vi "stage.vi"(8 "error in (no error)":errorcluster, 9 "stage number":u64, 11 "simonMessages in":refnum<class "simonMessages.lvclass">) -> (0 "error out":errorcluster, 3 "simonMessages out":refnum<class "simonMessages.lvclass">)   [LabVIEW 2019, in "simonMessages.lvclass"]
uses:
  simonMessages.lvclass
  simonMessages.lvclass/simonMessages.ctl
  TextDisplay/TextDisplay Class.lvclass
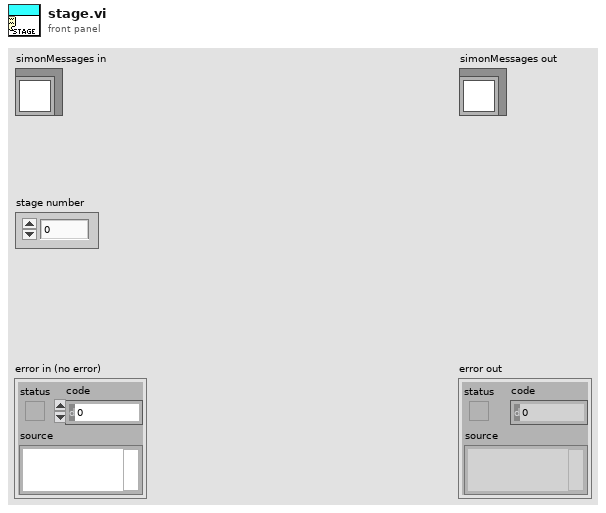
[diagram p1: front panel]
types:
  T1 = cluster{"Text":string, "Size":u8, "Justification":enum16{"Left", "Center", "Right"}, "Display Type":string}
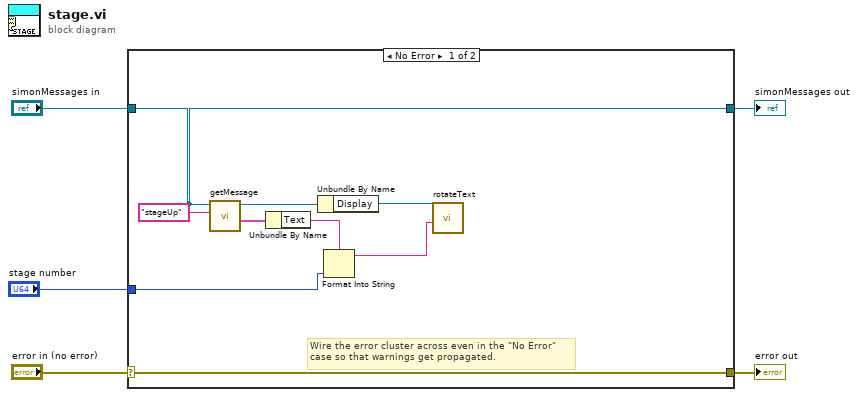
[diagram p0: block diagram]
diagram:
  n1 = case shown="No Error" "error in (no error)" {
    selector: "error in (no error)" -> [w14 w16]
    tunnel: [w14 w16] -> w4
    tunnel: [w12 w15] -> w2
    tunnel: "simonMessages in" -> [w12 w15]
    tunnel: "stage number" -> [w8 _]
    frame No Error {
      # "Wire the error cluster across even in the \"No Error\"\ncase so that warnings get propagated."
      n2 = call "getMessage.vi"("key"="stageUp", "simonMessages in"=w12) -> ("Message Cluster"=w9:T1, "simonMessages out"=w13:refnum<class "simonMessages.lvclass">)  [unwired: 7 in, 1 out]
      n3 = Unbundle By Name(w9) -> ("Text"=w6:string)
      n4 = Unbundle By Name(w13) -> ("Display"=w10:refnum<class "TextDisplay Class.lvclass">)
      n5 = Format Into String(format string=w6, w8) -> (resulting string=w7:string)  [unwired: 2 in, 1 out]
      n6 = call "rotateText.vi"("textIn"=w7, "TextDisplay Class in"=w10) -> ()  [unwired: 8 in, 2 out]
    }
    frame Error {
    }
  }
  "error out" <- w4
  "simonMessages out" <- w2
